vi "ADXL345 Accelerometer Test.vi"() -> ()   [LabVIEW 2015]
uses:
  <vilib>/MakerHub/LINX/Private/Type Defs/LINX Ref.ctl
  <vilib>/MakerHub/LINX/Private/Type Defs/Platform.ctl
  <vilib>/MakerHub/LINX/Private/Type Defs/Interface.ctl
  <vilib>/MakerHub/LINX/Private/Device/Type Defs/LINX Device Config.ctl
  <vilib>/MakerHub/LINX/Private/Device/Type Defs/TCP Config.ctl
  <vilib>/MakerHub/LINX/Private/Device/Type Defs/Channels.ctl
  <vilib>/MakerHub/LINX/Public/Sensors/Accelerometer/ADXL345/Address.ctl
  <vilib>/MakerHub/LINX/Private/Type Defs/User Platform.ctl
  <vilib>/MakerHub/LINX/LMH-LINX.lvlib
  <vilib>/MakerHub/LINX/Public/Sensors/Accelerometer/ADXL345/ADXL345.lvlib
  <vilib>/MakerHub/LINX/Private/Device/Device.lvlib
panel:
  out "Roll Pitch Yaw":T1
  out "Pitch":dbl(knob) scale=0.0..10.0
  out "Roll":dbl(knob) scale=-180.0..180.0
  out "G-Filtered":T1
  in  "alpha":dbl=0.5 format="%#_13g"
  in  "LINX Resource":T2
  in  "stop":bool
  out "Error Out":errorcluster
  in  "Serial Port":refnum<visa-resource-name>
  out "Device Name":string
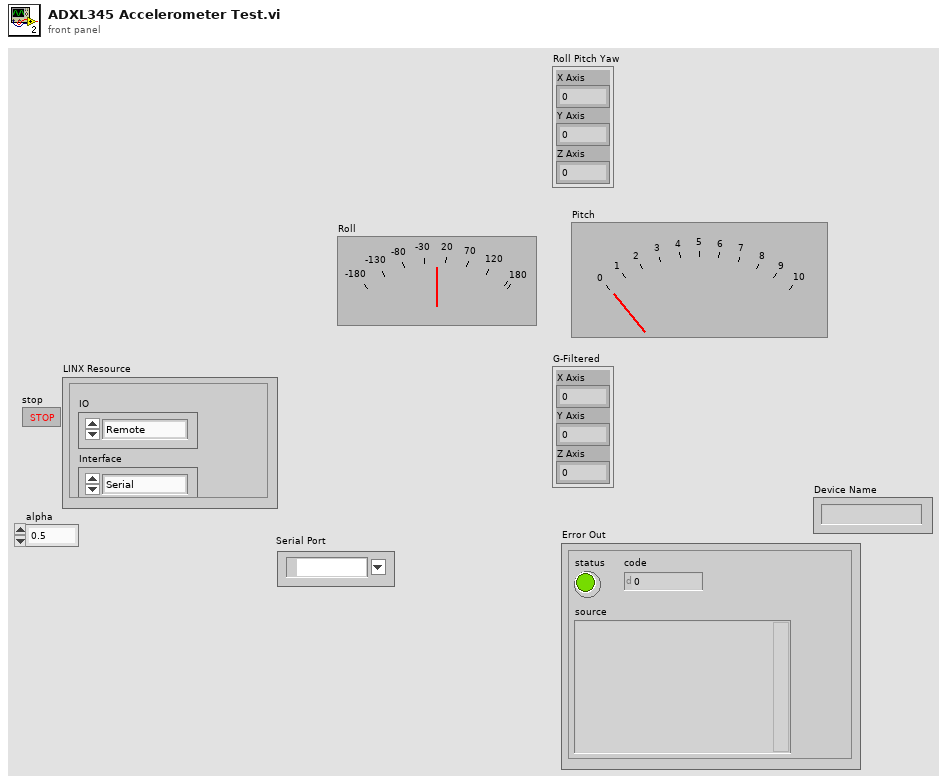
[diagram p1: front panel]
types:
  T1 = cluster{"X Axis":dbl, "Y Axis":dbl, "Z Axis":dbl}
  T2 = typedef "LMH-LINX.lvlib/LINX Ref.ctl" = cluster{"IO":T3, "Interface":T4, "LINX Device Config":T5}
  T3 = typedef "LMH-LINX.lvlib/Platform.ctl" = enum16{"Remote", "Local"}
  T4 = typedef "LMH-LINX.lvlib/Interface.ctl" = enum16{"Serial", "TCP"}
  T5 = typedef "LMH-LINX.lvlib/Device.lvlib/LINX Device Config.ctl" = cluster{"Interface":T4, "COM Port":refnum<visa-resource-name>, "TCP Configuration":T6, "Device Family":u8, "Device ID":u8, "Device Name":string, "TCP Ref":refnum<k5>, "Channels":T7}
  T6 = typedef "LMH-LINX.lvlib/Device.lvlib/TCP Config.ctl" = cluster{"IP Address":string, "Port":u16}
  T7 = typedef "LMH-LINX.lvlib/Channels.ctl" = cluster{"DI":u8[], "DO":u8[], "AI":u8[], "AO":u8[], "PWM":u8[], "QE":u8[], "UART":u8[], "I2C 2":u8[], "SPI":u8[], "CAN":u8[], "Servo":u8[], "AI Ref (V)":dbl, "AI Resolution (Bits)":u8, "AO Ref (V)":dbl, "AO Resolution (Bits)":u8}
  T8 = typedef "LMH-LINX.lvlib/User Platform.ctl" = enum16{"Default", "Remote", "Local"}
  T9 = typedef "LMH-LINX.lvlib/ADXL345.lvlib/Address.ctl" = enum16{"0x1D (ALT High)", "0x53 (ALT Low)"}
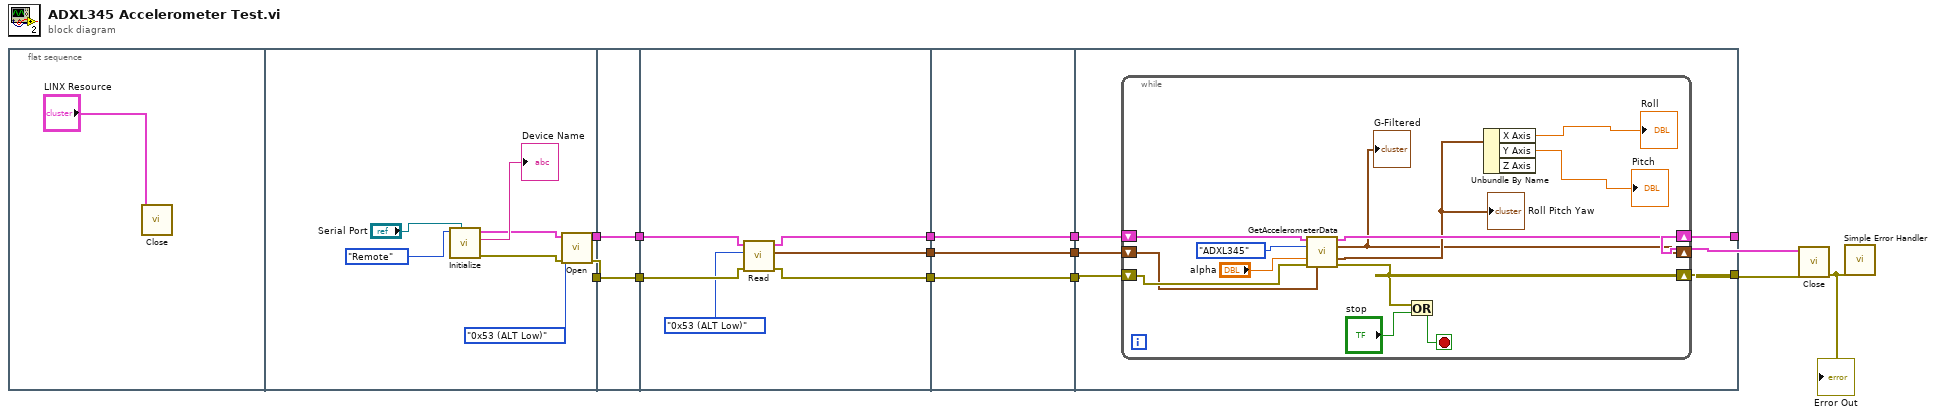
[diagram p0: block diagram]
diagram:
  n1 = flat-sequence {
    tunnel: [w19] -> w6
    tunnel: [w18] -> w4
    tunnel: w6 -> [w24]
    tunnel: [w24] -> w5
    tunnel: w4 -> [w23]
    tunnel: [w23] -> w3
    tunnel: w5 -> [w28]
    tunnel: [w29] -> w12
    tunnel: w3 -> [w27]
    tunnel: [w30] -> w10
    tunnel: [w26] -> w1
    tunnel: w12 -> [w33]
    tunnel: [w33] -> w11
    tunnel: w10 -> [w32]
    tunnel: [w32] -> w9
    tunnel: [w31] -> w2
    tunnel: w1 -> [w31]
    tunnel: w11 -> [w38]
    tunnel: w9 -> [w36]
    tunnel: [w37] -> w8
    tunnel: [w35] -> w7
    tunnel: w2 -> [w34]
    frame #0 {
      n2 = call <vilib>:"Close.vi"("LINX Resource"="LINX Resource") -> ()  [unwired: 10 in, 1 out]
    }
    frame #1 {
      n3 = call <vilib>:"Initialize.vi"("Serial Port"="Serial Port", "IO"=User_Platform."Remote" ("Platform")) -> ("Error Out"=w20:errorcluster, "Device Name"=→"Device Name":string, "LINX Resource"=w21:T2)  [unwired: 7 in]
      n4 = call <vilib>:"Open.vi"("Error In"=w20, "I2C Slave Address"=Address."0x53 (ALT Low)" ("ADXL345 Address"), "LINX Resource"=w21) -> ("Error Out"=w19:errorcluster, "LINX Resource"=w18:T2)  [unwired: 6 in, 1 out]
    }
    frame #2 {
    }
    frame #3 {
      n5 = call <vilib>:"Read.vi"("Error In"=w28, "I2C Slave Address"=Address."0x53 (ALT Low)" ("ADXL345 Address"), "LINX Resource"=w27) -> ("Error Out"=w29:errorcluster, "Acceleration Data (g)"=w26:T1, "LINX Resource"=w30:T2)  [unwired: 6 in]
    }
    frame #4 {
    }
    frame #5 {
      n6 = while {
        shift-right: [w46] -> w35
        shift-left: w38 -> [w47]
        shift-right: [w45] -> w37
        shift-left: w36 -> [w48]
        shift-right: [w39] -> _
        shift-left: w34 -> [w44]
        stop <- w50 stop-if-true
        n7 = call "GetAccelerometerData.vi"("LINX Resource"=w48, "Chip"=enum16{"LSM6DS1", "LSM6DS3", "ADXL345"}."ADXL345", "alpha"="alpha", "Error In"=w47, "input Gs"=w44) -> ("LINX Resource"=w45:T2, "Mag-Filtered"=w39:T1, "G-Filtered"=w43:T1, "Error Out"=w46:errorcluster)  [unwired: 6 in, 1 out]
        "G-Filtered" <- w39
        "Roll Pitch Yaw" <- w43
        n8 = Or(x=w46, y="stop") -> (x .or. y?=w50:bool)
        n9 = Unbundle By Name(w43) -> ("X Axis"=→"Roll":dbl, "Y Axis"=→"Pitch":dbl)  [unwired: 1 out]
      }
    }
  }
  n10 = call <vilib>:"Close.vi"("Error In"=w7, "LINX Resource"=w8) -> ("Error Out"=w13:errorcluster)  [unwired: 9 in]
  "Error Out" <- w13
  n11 = call <vilib>:"Simple Error Handler.vi"("error in (no error)"=w13) -> ()  [unwired: 4 in, 5 out]
